vi "write all relays.vi"(8 "error in (no error)":errorcluster, 10 "Boolean":bool, 11 "hardware in":refnum<class "hardware.lvclass">) -> (0 "error out":errorcluster, 3 "hardware out":refnum<class "hardware.lvclass">)   [LabVIEW 2025, in "hardware.lvclass"]
uses:
  hardware.lvclass
  hardware.lvclass/hardware.ctl
  <vilib>/DAQmx/write.llb/DAQmx Write (Digital 1D Bool 1Chan 1Samp).vi
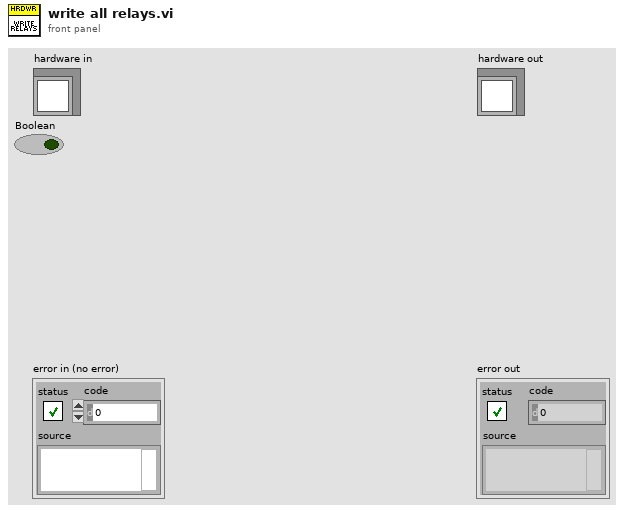
[diagram p1: front panel]
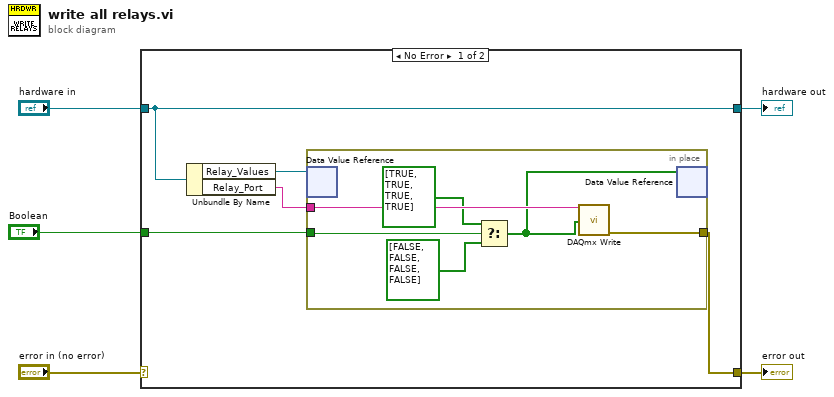
[diagram p0: block diagram]
diagram:
  n1 = case shown="No Error" "error in (no error)" {
    selector: "error in (no error)" -> [_ w18]
    tunnel: [w6 w18] -> w4
    tunnel: [w10 w17] -> w2
    tunnel: "hardware in" -> [w10 w17]
    tunnel: "Boolean" -> [w8 _]
    frame No Error {
      n2 = Unbundle By Name(w10) -> ("Relay_Values"=w9:refnum<data-value>, "Relay_Port"=w7:string)
      n3 = in-place {
        in-place-border: w8 -> [w15]
        in-place-border: w7 -> [w16]
        in-place-border: [w12] -> w6
        n4 = in-place-dvr #1(w9) -> ()  [unwired: 2 out]
        n5 = Select(t=bool[] [TRUE, TRUE, TRUE, TRUE] ("data value"), s=w15, f=bool[] [FALSE, FALSE, FALSE, FALSE] ("data value")) -> (s? t:f=w11:bool[])
        n6 = call-poly <vilib>:"DAQmx Write.vi"("task/channels in"=w16, "data"=w11) -> ("error out"=w12:errorcluster)  [unwired: 11 in, 2 out]
        n7 = in-place-dvr #1(w11) -> ()  [unwired: 2 out]
      }
    }
    frame Error {
    }
  }
  "error out" <- w4
  "hardware out" <- w2
